vi "Clean Up Structures.vi"(8 "error in (no error)":errorcluster, 11 "Block Diagram in":refnum<class "Block Diagram.lvclass">) -> (0 "error out":errorcluster, 3 "Block Diagram out":refnum<class "Block Diagram.lvclass">)   [LabVIEW 2015, in "Block Diagram.lvclass"]
uses:
  Block Diagram.lvclass
  Block Diagram.lvclass/Block Diagram.ctl
  Structures/Structures.lvclass/Structures.ctl
  Structures/Read Structure.vi
  Structures/Structures.lvclass
  Initial Sequence/Initial Sequence.lvclass
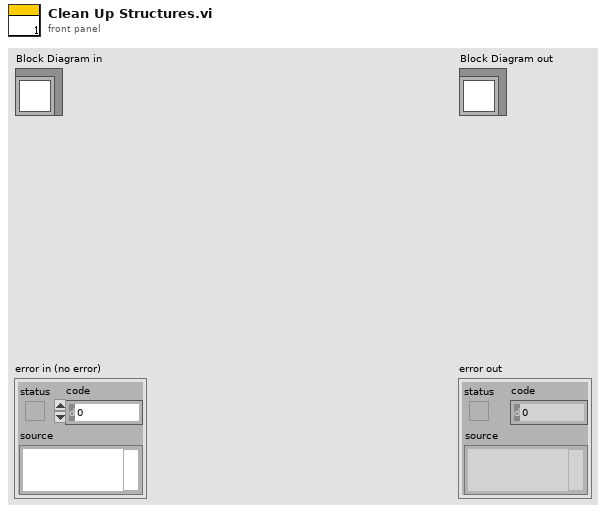
[diagram p1: front panel]
types:
  T1 = enum32{"Top Edges", "Vertical Centers", "Bottom Edges", "Left Edges", "Horizontal Centers", "Right Edges"}
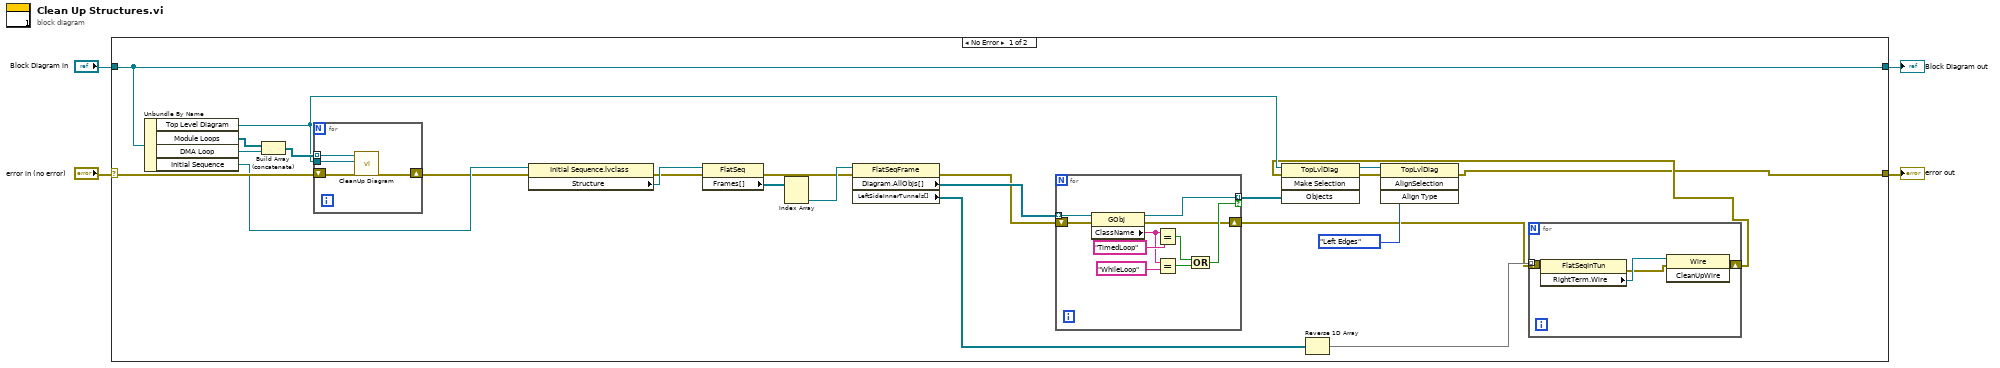
[diagram p0: block diagram]
diagram:
  n1 = case shown="No Error" "error in (no error)" {
    selector: "error in (no error)" -> [w27 w49]
    tunnel: [w5 w49] -> w3
    tunnel: [w28 w48] -> w1
    tunnel: "Block Diagram in" -> [w28 w48]
    frame No Error {
      n2 = Unbundle By Name(w28) -> ("Top Level Diagram"=w13:refnum<vi>, "Module Loops"=w25:refnum<class "Module Loop.lvclass">[], "DMA Loop"=w26:refnum<class "DMA Loop.lvclass">, "Initial Sequence"=w23:refnum<class "Initial Sequence.lvclass">)
      n3 = Build Array (concatenate)(w25, w26) -> (w24:refnum<class "Structures.lvclass">[])
      n4 = for {
        tunnel: w24 -> [w47] mode=indexing
        tunnel: w13 -> [w46]
        shift-right: [w44] -> w20
        shift-left: w27 -> [w45]
        n5 = call-dynamic "CleanUp Diagram.vi"("error in (no error)"=w45, "Top Level Diagram"=w46, "Structures in"=w47) -> ("error out"=w44:errorcluster)  [unwired: 7 in, 1 out]
      }
      n6 = property class="Initial Sequence.lvclass"(reference=w23, error in=w20) -> (error out=w19:errorcluster, "Structure"=w22:refnum<vi>)  [unwired: 1 out]
      n7 = property class="FlatSeq"(reference=w22, error in=w19) -> (error out=w14:errorcluster, "Frames[]"=w21:refnum<vi>[])  [unwired: 1 out]
      n8 = Index Array(array=w21) -> (element #2=w15:refnum<vi>)  [unwired: 2 in, 1 out]
      n9 = property class="FlatSeqFrame"(reference=w15, error in=w14) -> (error out=w10:errorcluster, "Diagram.AllObjs[]"=w12:refnum<vi>[], "LeftSideInnerTunnels[]"=w9:refnum<vi>[])  [unwired: 1 out]
      n10 = for {
        tunnel: w12 -> [w43] mode=indexing
        tunnel: [w38] -> w11 mode=indexing if=w37
        shift-right: [w35] -> w7
        shift-left: w10 -> [w36]
        n11 = property class="GObj"(reference=w43, error in=w36) -> (reference out=w38:refnum<vi>, error out=w35:errorcluster, "ClassName"=w34:string)
        n12 = Equal?(x=w34, y="TimedLoop") -> (x = y?=w41:bool)
        n13 = Equal?(x=w34, y="WhileLoop") -> (x = y?=w39:bool)
        n14 = Compound Arithmetic op=OR(w41, w39) -> (w37:bool)
      }
      n15 = Reverse 1D Array(array=w9) -> (reversed array=w8:refnum<vi>[])
      n16 = for {
        tunnel: w8 -> [w33] mode=indexing
        shift-right: [w29] -> w6
        shift-left: w7 -> [w32]
        n17 = property class="FlatSeqInTun"(reference=w33, error in=w32) -> (error out=w30:errorcluster, "RightTerm.Wire"=w31:refnum<vi>)  [unwired: 1 out]
        n18 = invoke class="Wire" method="CleanUpWire"(reference=w31, error in=w30) -> (error out=w29:errorcluster)  [unwired: 1 in, 2 out]
      }
      n19 = invoke class="TopLvlDiag" method="Make Selection"(reference=w13, error in=w6, "Objects"=w11) -> (reference out=w18:refnum<vi>, error out=w17:errorcluster)  [unwired: 1 in, 2 out]
      n20 = invoke class="TopLvlDiag" method="AlignSelection"(reference=w18, error in=w17, "Align Type"=T1."Left Edges") -> (error out=w5:errorcluster)  [unwired: 1 in, 3 out]
    }
    frame Error {
    }
  }
  "error out" <- w3
  "Block Diagram out" <- w1
